vi "新建数据文件夹.vi"   [LabVIEW 2020]
types:
  T1 = enum16{"open", "replace", "create", "open or create", "replace or create", "replace or create with confirmation"}
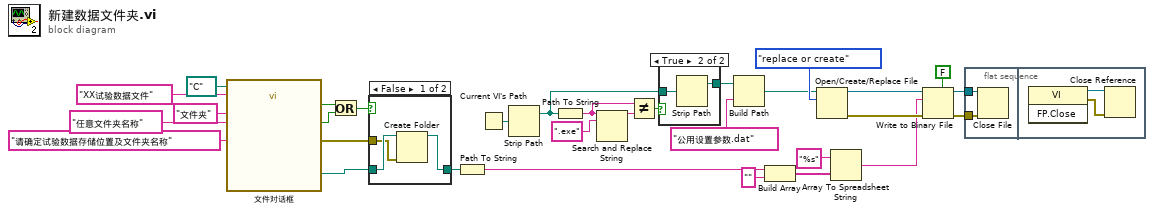
[diagram p0: block diagram]
diagram:
  n1 = call "文件对话框"("start path"=path "C:/", "prompt"="请确定试验数据存储位置及文件夹名称", "default name"="XX试验数据文件", "pattern (all files)"="文件夹", "pattern label"="任意文件夹名称") -> ("selected path"=w31:path, "exists"=w29:bool, "cancelled"=w27:bool, "error out"=w30:errorcluster)  [unwired: 7 in]
  n2 = Or(x=w29, y=w27) -> (x .or. y?=w28:bool)
  n3 = case shown="False" w28 {
    tunnel: w31 -> [w34 w35]
    tunnel: w30 -> [w33 _]
    tunnel: [w32 w35] -> w21
    frame False {
      n4 = Create Folder(path (use dialog)=w34, error in=w33) -> (created path=w32:path)  [unwired: 1 in, 2 out]
    }
    frame True {
    }
  }
  n5 = Path To String(path=w21) -> (string=w20:string)
  n6 = Current VI's Path() -> (path=w14:path)
  n7 = Strip Path(path=w14) -> (stripped path=w19:path)  [unwired: 1 out]
  n8 = Path To String(path=w19) -> (string=w17:string)
  n9 = Search and Replace String(input string=w17, search string=".exe" ("搜索字符串")) -> (result string=w16:string)  [unwired: 6 in, 3 out]
  n10 = Not Equal?(x=w17, y=w16) -> (x != y?=w18:bool)
  n11 = case shown="True" w18 {
    tunnel: w19 -> [w36 w38]
    tunnel: [w36 w37] -> w12
    frame False {
    }
    frame True {
      n12 = Strip Path(path=w38) -> (stripped path=w37:path)  [unwired: 1 out]
    }
  }
  n13 = Build Path(base path=w12, name or relative path="公用设置参数.dat") -> (appended path=w1:path)
  n14 = Build Array(w20, "" ("元素")) -> (w4:string[])
  n15 = Open/Create/Replace File(file path (use dialog)=w1, operation (0:open)=T1."replace or create" ("操作(0:open)")) -> (refnum out=w7:refnum<file>, error out=w6:errorcluster)  [unwired: 4 in, 1 out]
  n16 = Array To Spreadsheet String(array=w4, 3:"%s" ("format string")) -> (spreadsheet string=w2:string)  [unwired: 1 in]
  n17 = Write to Binary File(file (use dialog)=w7, data=w2, error in=w6, 5:FALSE ("预置数组或字符串大小？(T)")) -> (refnum out=w10:refnum<file>, error out=w9:errorcluster)  [unwired: 2 in, 1 out]
  n18 = flat-sequence {
    tunnel: w10 -> [w40]
    tunnel: w9 -> [w39]
    frame #0 {
      n19 = Close File(refnum=w40, error in=w39) -> ()  [unwired: 2 out]
    }
    frame #1 {
      n20 = invoke class="VI" method="FP.Close"() -> (reference out=w41:refnum<vi>, error out=w42:errorcluster)  [unwired: 3 in, 1 out]
      n21 = Close Reference(reference=w41, error in (no error)=w42) -> ()  [unwired: 1 out]
    }
  }
